vi "Compare.vi"(1 "RandomNumber":dbl, 2 "Guessed number":dbl) -> (0 "Output":dbl)   [LabVIEW 2021]
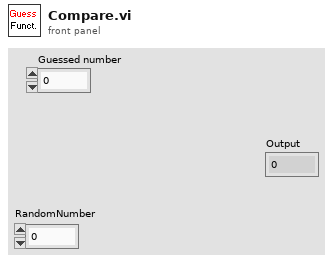
[diagram p1: front panel]
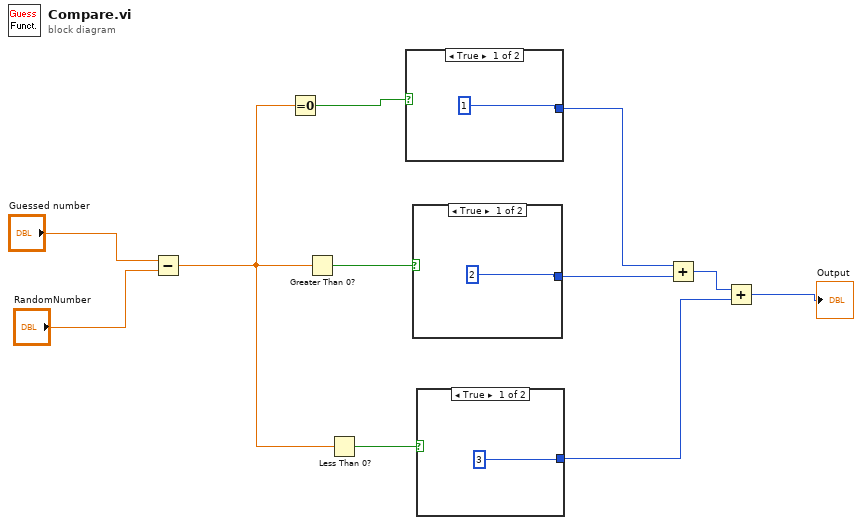
[diagram p0: block diagram]
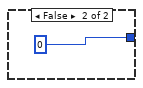
[diagram p2: hidden frame]
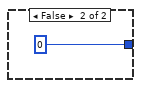
[diagram p3: hidden frame]
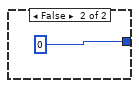
[diagram p4: hidden frame]
diagram:
  n1 = Subtract(x="Guessed number", y="RandomNumber") -> (x-y=w6:dbl)
  n2 = Equal To 0?(x=w6) -> (x = 0?=w9:bool)
  n3 = Greater Than 0?(x=w6) -> (x > 0?=w8:bool)
  n4 = Less Than 0?(x=w6) -> (x < 0?=w7:bool)
  n5 = case shown="True" w9 {
    tunnel: [1 0] -> w3
    frame True {
    }
    frame False {
    }
  }
  n6 = case shown="True" w8 {
    tunnel: [2 0] -> w4
    frame True {
    }
    frame False {
    }
  }
  n7 = case shown="True" w7 {
    tunnel: [3 0] -> w5
    frame True {
    }
    frame False {
    }
  }
  n8 = Add(x=w3, y=w4) -> (x+y=w2:i32)
  n9 = Add(x=w2, y=w5) -> (x+y=→"Output":i32)
